vi "GetConfigurationPagePath.vi"(8 "error in (no error)":errorcluster, 11 "IConfigurationPage in":refnum<class "IConfigurationPage.lvclass">) -> (0 "error out":errorcluster, 1 "Path":path, 3 "IConfigurationPage out":refnum<class "IConfigurationPage.lvclass">)   [LabVIEW 2020, in "ExtensionInterfaces.lvlib" / "IConfigurationPage.lvclass"]
uses:
  IConfigurationPage/IConfigurationPage.lvclass
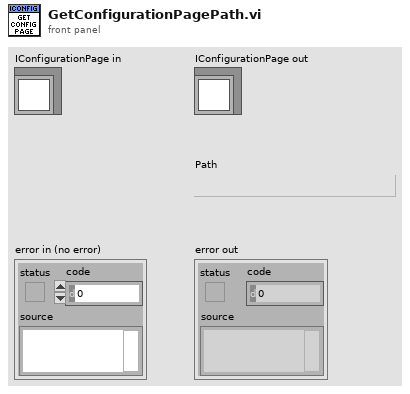
[diagram p1: front panel]
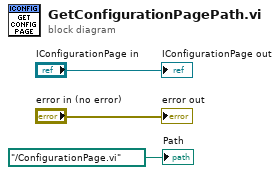
[diagram p0: block diagram]
diagram:
  "error out" <- "error in (no error)"
  "IConfigurationPage out" <- "IConfigurationPage in"
  "Path" <- path "../ConfigurationPage.vi" ("name or relative path")
